vi "Draw Terminal.vi"(5 "Center":i16=20, 7 "Index":i32, 10 "State":T1={"Worker Library Path"=path "", "Block Label"="", "Types"=[], "Selections"=[], "Icon"={"image type"=0, "image depth"=0, "image"=[], "mask"=[], "colors"=[], "Rectangle"={"left"=0, "top"=0, "right"=0, "bottom"=0}}, "Errors"={"Terminals"=[], "Generate"={"status"=FALSE, "code"=0, "source"=""}}, "Calculated Sizes"={"Block Width"=100, "Block Height"=0, "Half Width"=0, "Icon Top"=0, "Icon Bottom"=0, "Label Width"=0, "Half Label"=0, "Label Top"=0, "Text Width"=0, "Half Text"=0, "Text Height"=0, "Label Height"=0, "Expanded Width"=0, "Label Bottom"=0, "Expanded Top"=0, "Expanded Bottom"=0, "Expanded Height"=0, "Min Height"=0, "Max Height"=0}, "Special Terminal Indices"={"Action"=-1, "Init"=-1, "Tag"=-1, "State in"=-1, "State out"=-1, "Error"=-1}, "Terminals"=[]}, 11 "Picture In":picture) -> (3 "Picture":picture)   [LabVIEW 2022 SP3, in "FlexBlocks Support.lvlib"]
uses:
  FlexBlocks Support.lvlib
  Flex Block/State.ctl
  Type Descriptor.ctl
  Terminal Direction.ctl
  Value Mode.ctl
  Special Terminal.ctl
  <vilib>/picture/picture.llb/imagedata.ctl
  XNode Errors.ctl
  Calculated Sizes.ctl
  Special Terminal Indices.ctl
  Terminal Status.ctl
  Terminal State.ctl
  Terminal Draw Style.ctl
  Flex Block/Flex Block.xnode
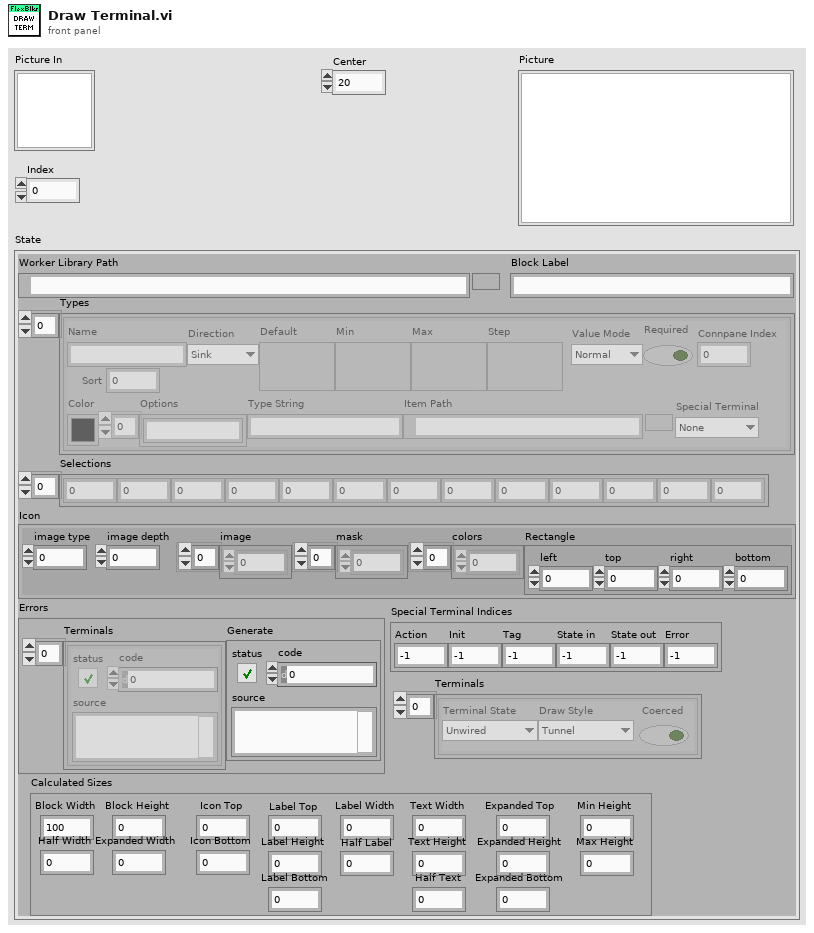
[diagram p1: front panel]
types:
  T1 = typedef "Flex Block.xnode/State.ctl" = cluster{"Worker Library Path":path, "Block Label":string, "Types":T2[], "Selections":i32[], "Icon":T6, "Errors":T7, "Calculated Sizes":T8, "Special Terminal Indices":T9, "Terminals":T10[]}
  T2 = typedef "FlexBlocks Support.lvlib/Type Descriptor.ctl" = cluster{"Name":string, "Direction":T3, "Default":variant, "Min":variant, "Max":variant, "Step":variant, "Value Mode":T4, "Color":u32, "Options":string[], "Type String":string, "Item Path":path, "Required":bool, "Connpane Index":i32, "Special Terminal":T5, "Sort":i32}
  T3 = typedef "FlexBlocks Support.lvlib/Terminal Direction.ctl" = enum16{"Sink", "Source"}
  T4 = typedef "FlexBlocks Support.lvlib/Value Mode.ctl" = enum16{"Normal", "Range", "Select"}
  T5 = typedef "FlexBlocks Support.lvlib/Special Terminal.ctl" = enum16{"None", "Action", "Init", "Tag", "State in", "State out", "Error"}
  T6 = typedef "imagedata.ctl" = cluster{"image type":i32, "image depth":i32, "image":u8[], "mask":u8[], "colors":u32[], "Rectangle":cluster{"left":i16, "top":i16, "right":i16, "bottom":i16}}
  T7 = typedef "FlexBlocks Support.lvlib/XNode Errors.ctl" = cluster{"Terminals":errorcluster[], "Generate":errorcluster}
  T8 = typedef "FlexBlocks Support.lvlib/Calculated Sizes.ctl" = cluster{"Block Width":i32, "Block Height":i32, "Half Width":i32, "Icon Top":i32, "Icon Bottom":i32, "Label Width":i32, "Half Label":i32, "Label Top":i32, "Text Width":i32, "Half Text":i32, "Text Height":i32, "Label Height":i32, "Expanded Width":i32, "Label Bottom":i32, "Expanded Top":i32, "Expanded Bottom":i32, "Expanded Height":i32, "Min Height":i32, "Max Height":i32}
  T9 = typedef "FlexBlocks Support.lvlib/Special Terminal Indices.ctl" = cluster{"Action":i32, "Init":i32, "Tag":i32, "State in":i32, "State out":i32, "Error":i32}
  T10 = typedef "FlexBlocks Support.lvlib/Terminal Status.ctl" = cluster{"Terminal State":T11, "Draw Style":T12, "Coerced":bool}
  T11 = typedef "FlexBlocks Support.lvlib/Terminal State.ctl" = enum16{"Unwired", "BadType", "BadRef", "Channel", "Value", "Control Ref"}
  T12 = typedef "FlexBlocks Support.lvlib/Terminal Draw Style.ctl" = enum16{"Tunnel", "BadType", "BadRef", "Channel", "Value", "Control Ref"}
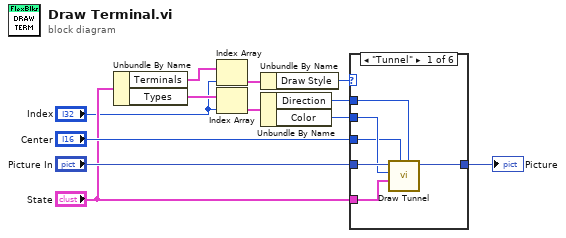
[diagram p0: block diagram]
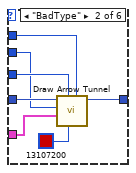
[diagram p2: hidden frame]
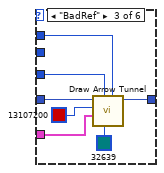
[diagram p3: hidden frame]
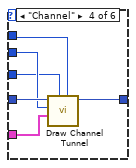
[diagram p4: hidden frame]
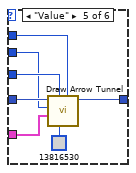
[diagram p5: hidden frame]
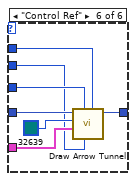
[diagram p6: hidden frame]
diagram:
  n1 = Unbundle By Name("State") -> ("Terminals"=w8:T10[], "Types"=w6:T2[])
  n2 = Index Array(array=w8, index="Index") -> (element=w7:T10)
  n3 = Index Array(array=w6, index="Index") -> (element=w4:T2)
  n4 = Unbundle By Name(w7) -> ("Draw Style"=w12:T12)
  n5 = Unbundle By Name(w4) -> ("Direction"=w2:T3, "Color"=w3:u32)
  n6 = case shown="\"Tunnel\"" w12 {
    tunnel: "Picture In" -> [w18 w25 w32 w38 w45 w52]
    tunnel: "State" -> [w17 w21 w30 w34 w39 w48]
    tunnel: "Center" -> [w15 w24 w28 w33 w43 w51]
    tunnel: w3 -> [w16 w19 _ w35 w41 w47]
    tunnel: w2 -> [w14 w23 w27 w36 w42 w50]
    tunnel: [w13 w22 w26 w37 w44 w46] -> w1
    frame "Tunnel" {
      n7 = call "Draw Tunnel.vi"("Direction"=w14, "Center"=w15, "State"=w17, "Center Color"=w16, "Picture In"=w18) -> ("Picture"=w13:picture)  [unwired: 6 in]
    }
    frame "BadType" {
      n8 = call "Draw Arrow Tunnel.vi"("Direction"=w23, "Outer Color"=u32 13107200 ("Arrow Color"), "Center"=w24, "State"=w21, "Arrow Color"=w19, "Picture In"=w25) -> ("Picture"=w22:picture)  [unwired: 5 in]
    }
    frame "BadRef" {
      n9 = call "Draw Arrow Tunnel.vi"("Direction"=w27, "Outer Color"=u32 32639, "Center"=w28, "State"=w30, "Arrow Color"=u32 13107200, "Picture In"=w32) -> ("Picture"=w26:picture)  [unwired: 5 in]
    }
    frame "Channel" {
      n10 = call "Draw Channel Tunnel.vi"("Direction"=w36, "Center"=w33, "State"=w34, "Type Color"=w35, "Picture In"=w38) -> ("Picture"=w37:picture)  [unwired: 6 in]
    }
    frame "Value" {
      n11 = call "Draw Arrow Tunnel.vi"("Direction"=w42, "Outer Color"=u32 13816530, "Center"=w43, "State"=w39, "Arrow Color"=w41, "Picture In"=w45) -> ("Picture"=w44:picture)  [unwired: 5 in]
    }
    frame "Control Ref" {
      n12 = call "Draw Arrow Tunnel.vi"("Direction"=w50, "Outer Color"=w47, "Center"=w51, "State"=w48, "Arrow Color"=u32 32639, "Picture In"=w52) -> ("Picture"=w46:picture)  [unwired: 5 in]
    }
  }
  "Picture" <- w1
